vi "tkrsa6100 Config RF Input.vi"(0 "VISA Resource Name":refnum<visa-resource-name>, 1 "RF Atten (dB)(0)":T2(ring), 5 "Set/Read\nInput Setting (SET)":enum16{"SET", "READ"}(ring), 7 "Input Settings\n(REFERENCE LEVEL)":T3(ring), 9 "Ref Level (0)":dbl, 11 "error in (no error)":errorcluster, 12 "Vertical Units (DBM)":T1(ring)) -> (4 "dup VISA Resource Name":refnum<visa-resource-name>, 6 "Input Setting\nResponse String":string, 15 "error out":errorcluster {"code" format="%#.0f"})   [LabVIEW 2020, in "Library Instrument & Equipement.lvlib" / "Library Spectrum Analyser.lvlib"]
doc: "Prerequisites for use:\n \nThis VI is valid in all measurement views.\n\nThis VI controls the following functions:\nSets/reads the Reference Level.\nSets/reads the RF Attenuation.\nSets/reads the status of the Auto Attenuation function.\nSets/reads whether the Preamp is enabled or disabled.\nSets/reads the vertical scale units.\n\nerror in (no error) is checked by tkrsa6100 Write/Read wError Query.vi for any pending errors.\n\nIf error in status is ERROR:\n\nerror in (no error) and VISA Resource Name are passed straight through to error out and dup VISA Resource Name of the Write/Read Drivers and returned to the calling function. No commands are processed.\n\nIf error in status is NO ERROR:\n\nBy passing SET to Set/Read Input Settings (SET) the following parameters can be written. Pass the desired parameter to Input Setting (REFERENCE LEVEL). Additional parameters to be passed are specified with each function.\n\nOne command/query is executed per VI call.\n\nREFERENCE LEVEL\nControls the instrument Reference Level (top of screen amplitude). Pass the desired level in the current vertical scale units to numeric control Reference Level (0). The vertical units can be changed with the VERTICAL UNITS function in this VI.\n\nRF ATTENUATION\nControls the RF Attenuation. Pass the desired attenuation to enumerated control RF Attenuation (0).\n\nAUTO ATTENUATION ON\nAUTO ATTENUATION OFF\nControls the auto attenuation function. No further parameters are necessary to be passed.\n\nPREAMP ON\nPREAMP OFF\nControls whether or not to use the input preamplifier. No further parameters are necessary to be passed.\n\nVERTICAL UNITS\nSelects the vertical scale units. Pass the desired selection to enumerated control Vertical Units (dBm).\n\nThe following parameters can be read by passing READ to enumerated control Set/Read Input Settings (SET) and the parameter to be read to Input Setting (REFERENCE LEVEL). The current values are returned in string indicator Input Settings Response String.\n\nREFERENCE LEVEL\nReturns the current reference level in the current vertical scale units.\n\nValid Return Values\n\nRange varies with the vertical scale units setting\n\nMajor unit settings ranges are:\n\ndBm -170 to +50dBm\nVolts 1e-9 to 70.7107 volts\nWatts 10e-21 to 100 watts\nAmps 14.14e-12 to 1.414\n\nRF ATTENUATION\nValid return values are 0 to 75dB in 5dB steps.\n\nAUTO ATTENUATION ON\nAUTO ATTENUATION OFF\nEither selection queries the status of the auto attenuation function.\nValid return values are \n0 (off)\n1(on)\n\nPREAMP ON\nPREAMP OFF\nEither selection queries the status of the preamp.\nValid return values are \n0 (Off)\n1 (On)\n\nVERTICAL UNITS\nReturns the current vertical scale units setting.\n\nValid return values are:\n\nDBM\nVOLT\nDBUV (dBuV)\nDBMV (dBmV)\nDBV (dBV)\nWATT\nDBUW (dBuW)\nDBW (dBW)\nAMPS\nDBUA (dBuA)\nDBUV_M (dBuV/Meter)\nDBUA_M (dBuA/Meter)\n\nThe appropriate command/query string is passed to tkrsa6100 Write/Read wError Query.vi. Input Error Query? is unwired so query SYST:ERR? is appended to the command string and any current error information is displayed in cluster Error Out.\nOn completion dup VISA Resource Name, Error Out, and Input Settings Response String are returned to the calling function."
uses:
  Library Spectrum Analyser.lvlib
panel:
  # "RSA6100 Config RF Input Settings Driver"
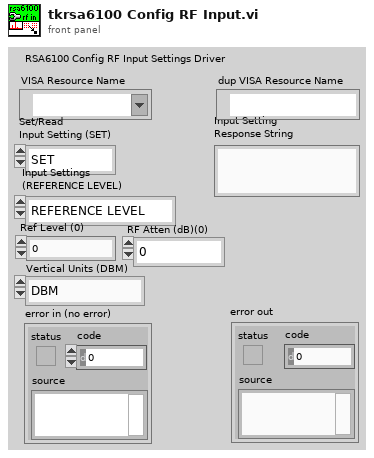
[diagram p1: front panel]
types:
  T1 = enum16{"DBM", "VOLTS", "DBUV", "DBMV", "DBV", "WATTS", "DBUW", "DBW", "AMPS", "DBUA", "DBUV/M", "DBUA/M"}
  T2 = enum16{"0", "5", "10", "15", "20", "25", "30", "35", "40", "45", "50", "55", "60", "65", "70", "75"}
  T3 = enum16{"REFERENCE LEVEL", "RF ATTENUATION", "AUTO ATTENUATION ON", "AUTO ATTENUATION OFF", "PREAMP ON", "PREAMP OFF", "VERTICAL UNITS"}
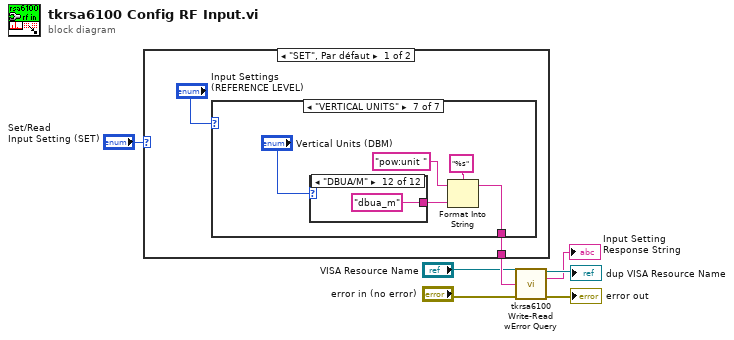
[diagram p0: block diagram]
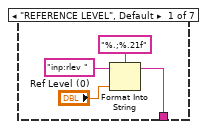
[diagram p2: hidden frame]
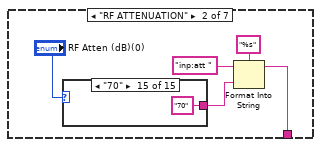
[diagram p3: hidden frame]
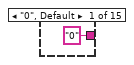
[diagram p4: hidden frame]
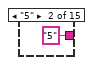
[diagram p5: hidden frame]
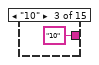
[diagram p6: hidden frame]
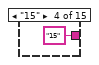
[diagram p7: hidden frame]
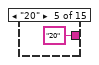
[diagram p8: hidden frame]
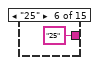
[diagram p9: hidden frame]
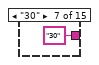
[diagram p10: hidden frame]
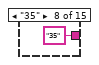
[diagram p11: hidden frame]
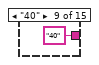
[diagram p12: hidden frame]
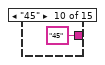
[diagram p13: hidden frame]
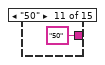
[diagram p14: hidden frame]
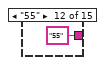
[diagram p15: hidden frame]
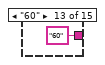
[diagram p16: hidden frame]
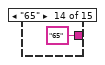
[diagram p17: hidden frame]
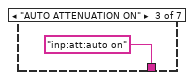
[diagram p18: hidden frame]
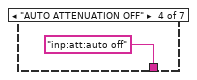
[diagram p19: hidden frame]
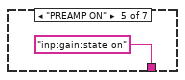
[diagram p20: hidden frame]
diagram:
  n1 = case shown="\"SET\", Par défaut" "Set/Read\nInput Setting (SET)" {
    tunnel: [w9 w56] -> w4
    frame "SET", Default {
      n2 = case shown="\"VERTICAL UNITS\"" "Input Settings\n(REFERENCE LEVEL)" {
        tunnel: [w12 w17 "inp:att:auto on" ("Command") "inp:att:auto off" ("Command") "inp:gain:state on" ("Command") "inp:gain:state off" ("Command") w41] -> w9
        frame "REFERENCE LEVEL", Default {
          n3 = Format Into String(format string="%.;%.21f", initial string="inp:rlev " ("Command"), "Ref Level (0)") -> (resulting string=w12:string)  [unwired: 1 in, 1 out]
        }
        frame "RF ATTENUATION" {
          n4 = case shown="\"70\"" "RF Atten (dB)(0)" {
            tunnel: ["0" ("Command") "5" ("Command") "10" ("Command") "15" ("Command") "20" ("Command") "25" ("Command") "30" ("Command") "35" ("Command") "40" ("Command") "45" ("Command") "50" ("Command") "55" ("Command") "60" ("Command") "65" ("Command") "70" ("Command")] -> w14
            frame "0", Default {
            }
            frame "5" {
            }
            frame "10" {
            }
            frame "15" {
            }
            frame "20" {
            }
            frame "25" {
            }
            frame "30" {
            }
            frame "35" {
            }
            frame "40" {
            }
            frame "45" {
            }
            frame "50" {
            }
            frame "55" {
            }
            frame "60" {
            }
            frame "65" {
            }
            frame "70" {
            }
          }
          n5 = Format Into String(format string="%s", initial string="inp:att " ("Command"), w14) -> (resulting string=w17:string)  [unwired: 1 in, 1 out]
        }
        frame "AUTO ATTENUATION ON" {
        }
        frame "AUTO ATTENUATION OFF" {
        }
        frame "PREAMP ON" {
        }
        frame "PREAMP OFF" {
        }
        frame "VERTICAL UNITS" {
          n6 = case shown="\"DBUA/M\"" "Vertical Units (DBM)" {
            tunnel: ["dbm" ("Command") "volt" ("Command") "dbuv" ("Command") "dbmv" ("Command") "dbv" ("Command") "watt" ("Command") "dbuw" ("Command") "dbw" ("Command") "amps" ("Command") "dbua" ("Command") "dbuv_m" ("Command") "dbua_m" ("Command")] -> w38
            frame "DBM", Default {
            }
            frame "VOLTS" {
            }
            frame "DBUV" {
            }
            frame "DBMV" {
            }
            frame "DBV" {
            }
            frame "WATTS" {
            }
            frame "DBUW" {
            }
            frame "DBW" {
            }
            frame "AMPS" {
            }
            frame "DBUA" {
            }
            frame "DBUV/M" {
            }
            frame "DBUA/M" {
            }
          }
          n7 = Format Into String(format string="%s", initial string="pow:unit " ("Command"), w38) -> (resulting string=w41:string)  [unwired: 1 in, 1 out]
        }
      }
    }
    frame "READ" {
      n8 = local read "Input Settings\n(REFERENCE LEVEL)"() -> (w55:T3)
      n9 = case shown="\"REFERENCE LEVEL\"" w55 {
        tunnel: ["inp:rlev?" ("Command") "inp:att:auto?" ("Command") "inp:att:auto?" ("Command") "pow:unit?" ("Command") "input:att?" ("Command") "inp:gain:state?" ("Command") "inp:gain:state?" ("Command")] -> w56
        frame "REFERENCE LEVEL" {
        }
        frame "AUTO ATTENUATION OFF" {
        }
        frame "AUTO ATTENUATION ON" {
        }
        frame "VERTICAL UNITS" {
        }
        frame "RF ATTENUATION" {
        }
        frame "PREAMP OFF" {
        }
        frame "PREAMP ON" {
        }
      }
    }
  }
  n10 = call "tkrsa6100 Write-Read wError Query.vi"("VISA Resource Name"="VISA Resource Name", "Command (Empty String)"=w4, "error in (no error)"="error in (no error)") -> ("dup VISA Resource Name"=→"dup VISA Resource Name":refnum<visa-resource-name>, "Response"=→"Input Setting\nResponse String":string, "error out"=→"error out":errorcluster)  [unwired: 4 in, 6 out]
